vi "Get Position For Align Or Distribute.vi"(8 "Error In":errorcluster, 10 "Vertical? (F: Horizontal)":bool, 11 "Panel Object in":refnum<class "Panel Object.lvclass">) -> (0 "Error Out":errorcluster, 1 "Position":i32, 2 "Applicable?":bool, 3 "Panel Object out":refnum<class "Panel Object.lvclass">)   [LabVIEW 2017, in "Panel Object.lvclass"]
uses:
  Panel Object.lvclass
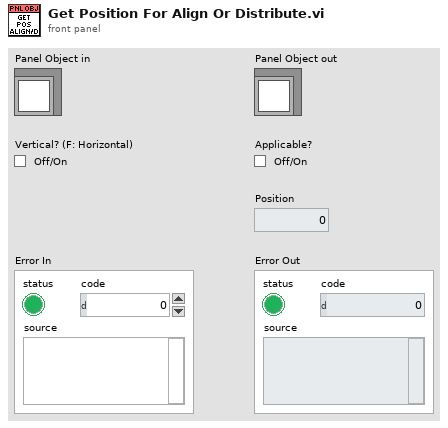
[diagram p1: front panel]
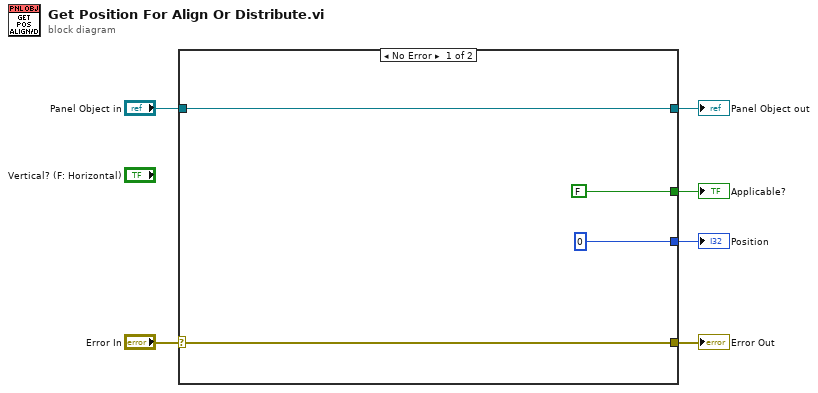
[diagram p0: block diagram]
diagram:
  n1 = case shown="No Error" "Error In" {
    selector: "Error In" -> [w9 w12]
    tunnel: [w9 w12] -> w3
    tunnel: [w10 w11] -> w5
    tunnel: "Panel Object in" -> [w10 w11]
    tunnel: [FALSE _] -> w2
    tunnel: [0 ("Position") _] -> w1
    frame No Error {
    }
    frame Error {
    }
  }
  "Panel Object out" <- w5
  "Error Out" <- w3
  "Applicable?" <- w2
  "Position" <- w1
